vi "Project Reference.vi"(8 "error in (no error)":errorcluster) -> (0 "error out":errorcluster, 3 "prj ref":refnum<vi>)   [LabVIEW 2014, in "lvprj2html.lvlib"]
uses:
  lvprj2html.lvlib
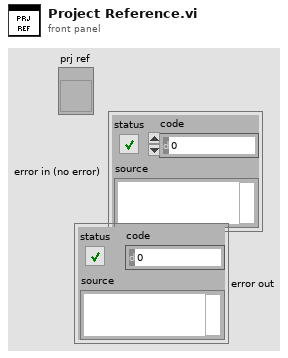
[diagram p1: front panel]
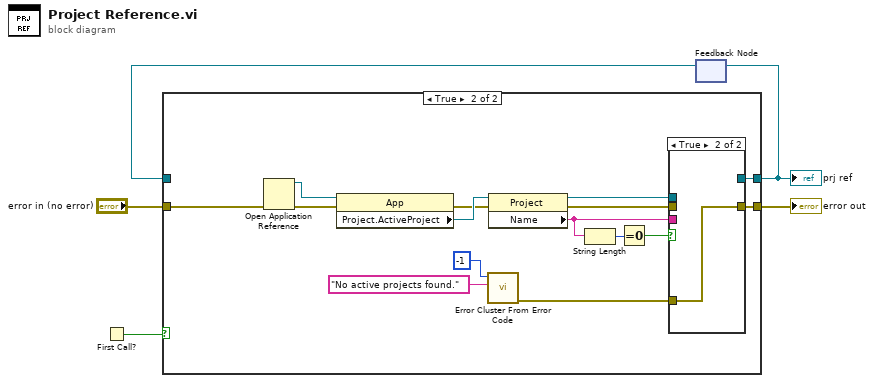
[diagram p0: block diagram]
diagram:
  n1 = First Call?() -> (First Call?: T/F=w3:bool)
  n2 = feedback #1() -> (w1:refnum<vi>)  [unwired: 1 in]
  n3 = case shown="True" w3 {
    tunnel: "error in (no error)" -> [w7 w8]
    tunnel: [w7 w17] -> w4
    tunnel: [w6 w16] -> w2
    tunnel: w1 -> [w6 _]
    frame False {
    }
    frame True {
      n4 = Open Application Reference(8:w8) -> (0:w9:errorcluster, 3:w10:refnum<vi>)  [unwired: 3 in]
      n5 = property class="App"(reference=w10, error in=w9) -> (error out=w20:errorcluster, "Project.ActiveProject"=w22:refnum<vi>)  [unwired: 1 out]
      n6 = call <vilib>:"Error Cluster From Error Code.vi"("error message (\"\")"="No active projects found." ("source"), "error code (0)"=-1) -> ("error out"=w11:errorcluster)  [unwired: 7 in]
      n7 = property class="Project"(reference=w22, error in=w20) -> (reference out=w15:refnum<vi>, error out=w18:errorcluster, "Name"=w14:string)
      n8 = String Length(string=w14) -> (length=w21:i32)
      n9 = Equal To 0?(x=w21) -> (x = 0?=w19:bool)
      n10 = case shown="True" w19 {
        tunnel: w18 -> [w23 _]
        tunnel: [w23 w25] -> w17
        tunnel: [w24 _] -> w16
        tunnel: w15 -> [w24 _]
        tunnel: w11 -> [_ w25]
        tunnel: w14 -> [_ _]
        frame False {
        }
        frame True {
        }
      }
    }
  }
  "prj ref" <- w2
  "error out" <- w4
  n11 = feedback-in #1(w2) -> ()
